vi "MyInterfaceMethod.vi"(0 "reference in":refnum<class "MyClass2_IMyInterface.lvclass">, 1 "MyParameter":dbl, 5 "error in (no error)":errorcluster) -> (14 "reference out":refnum<class "MyClass2_IMyInterface.lvclass">, 19 "error out":errorcluster)   [LabVIEW 2020, in "MyClass2_IMyInterface.lvclass"]
uses:
  MyClass2_IMyInterface.lvclass
  MyClass2.lvclass
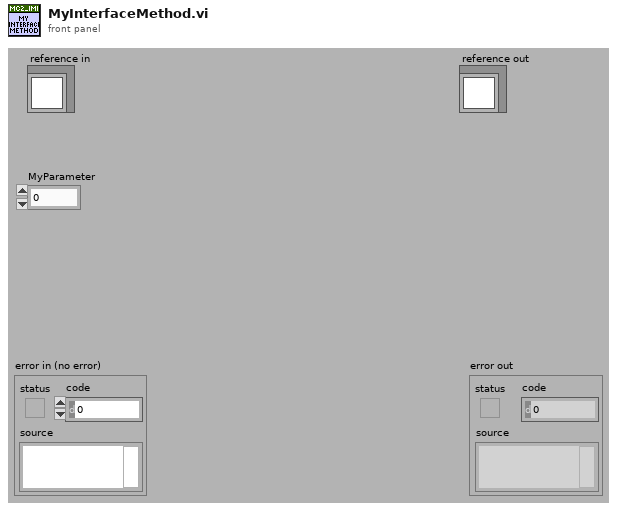
[diagram p1: front panel]
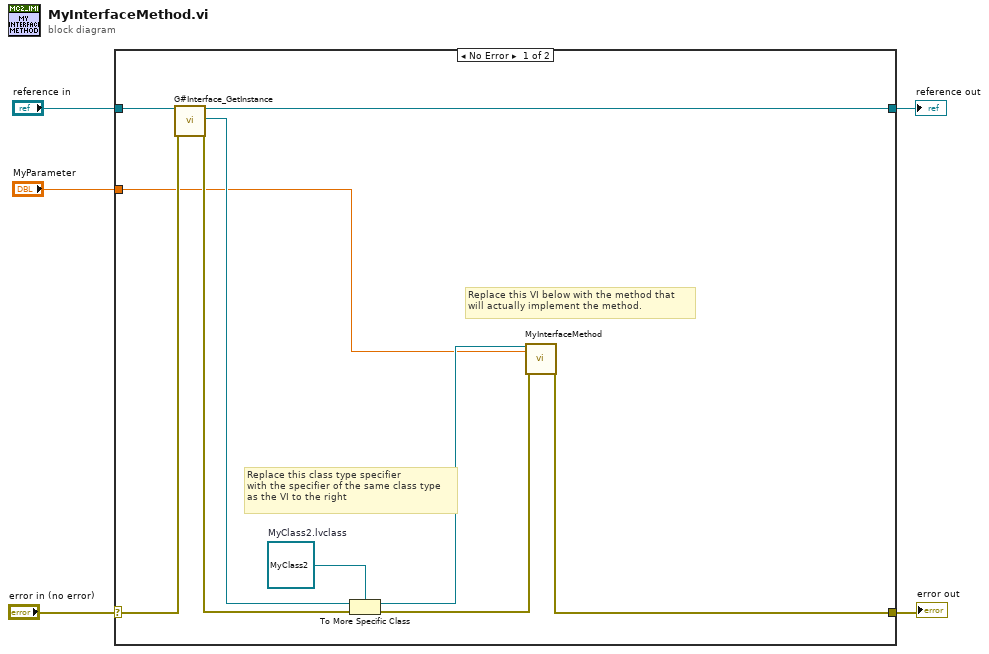
[diagram p0: block diagram]
diagram:
  n1 = case shown="No Error" "error in (no error)" {
    selector: "error in (no error)" -> [w13 w17]
    tunnel: [w9 w17] -> w4
    tunnel: [w14 w16] -> w2
    tunnel: "reference in" -> [w15 w16]
    tunnel: "MyParameter" -> [w6 _]
    frame No Error {
      w8 = refnum<class "MyClass2.lvclass"> refnum  # MyClass2.lvclass
      # "Replace this class type specifier\nwith the specifier of the same class type\nas the VI to the right"
      # "Replace this VI below with the method that\nwill actually implement the method."
      n2 = call-dynamic "G#Interface_GetInstance.vi"("reference in"=w15, "error in (no error)"=w13) -> ("reference out"=w14:refnum<class "MyClass2_IMyInterface.lvclass">, "G#Object"=w11:refnum<class "G#Object.lvclass">, "error out"=w12:errorcluster)  [unwired: 14 in, 1 out]
      n3 = To More Specific Class(target class=w8, reference=w11, error in=w12) -> (specific class reference=w7:refnum<class "MyClass2.lvclass">, error out=w10:errorcluster)
      n4 = call-dynamic "MyInterfaceMethod.vi"("reference in"=w7, "MyParameter"=w6, "error in (no error)"=w10) -> ("error out"=w9:errorcluster)  [unwired: 15 in, 1 out]
    }
    frame Error {
    }
  }
  "error out" <- w4
  "reference out" <- w2
